vi "Package List to Files and Library Package List.vi"(8 "error in (no error)":errorcluster, 10 "Packages":string[](array[string])) -> (0 "error out":errorcluster, 2 "Library Packages":string[](array[string]), 3 "File Packages":string[](array[string]))   [LabVIEW 2015, in "G CLI VIP.lvlib"]
uses:
  G CLI VIP.lvlib
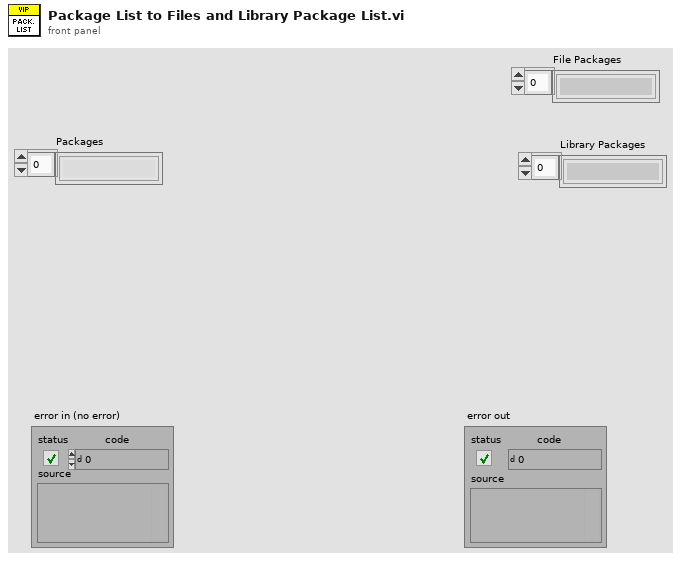
[diagram p1: front panel]
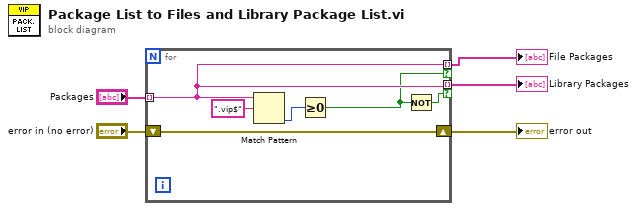
[diagram p0: block diagram]
diagram:
  n1 = for {
    tunnel: "Packages" -> [w8] mode=indexing
    shift-right: [w11] -> w3
    shift-left: "error in (no error)" -> [w11]
    tunnel: [w8] -> w1 mode=indexing if=w6
    tunnel: [w8] -> w2 mode=indexing if=w7
    n2 = Match Pattern(string=w8, regular expression=".vip$") -> (offset past match=w9:i32)  [unwired: 1 in, 3 out]
    n3 = Greater Or Equal To 0?(x=w9) -> (x >= 0?=w6:bool)
    n4 = Not(x=w6) -> (.not. x?=w7:bool)
  }
  "error out" <- w3
  "File Packages" <- w1
  "Library Packages" <- w2
